vi "DisplayLogic_DrawPressStart.vi"(0 "Player":u8, 1 "ActivePixel":cluster{"h_pixel":i16, "v_pixel":i16}, 4 "PressStartPos":T1) -> (15 "PixelData":bool[](array[boolean]), 18 "Draw":bool)   [LabVIEW 2018]
uses:
  Control_GameOverGlobal.vi
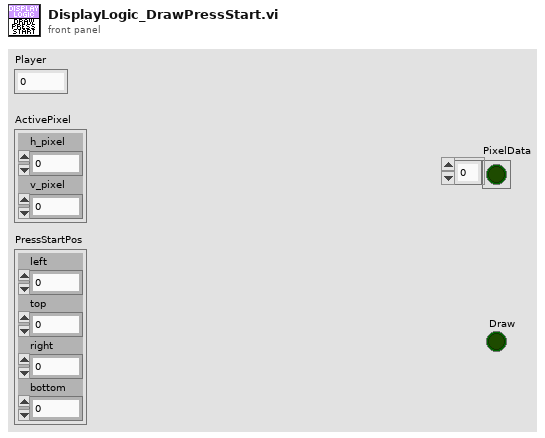
[diagram p1: front panel]
types:
  T1 = cluster{"left":i16, "top":i16, "right":i16, "bottom":i16}
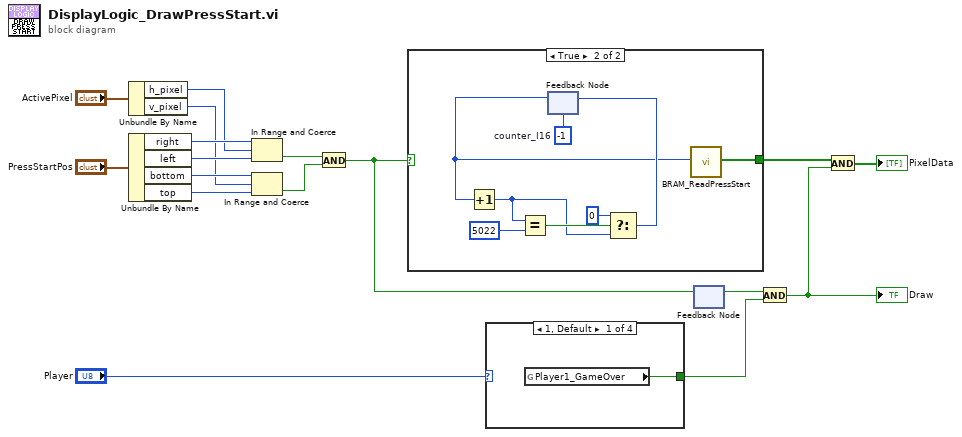
[diagram p0: block diagram]
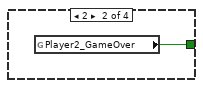
[diagram p2: hidden frame]
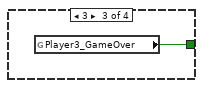
[diagram p3: hidden frame]
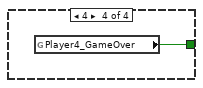
[diagram p4: hidden frame]
diagram:
  n1 = Unbundle By Name("ActivePixel") -> ("h_pixel"=w9:i16, "v_pixel"=w8:i16)
  n2 = Unbundle By Name("PressStartPos") -> ("right"=w13:i16, "left"=w17:i16, "bottom"=w11:i16, "top"=w14:i16)
  n3 = In Range and Coerce(upper limit=w13, x=w9, lower limit=w17) -> (In Range?=w16:bool)  [unwired: 1 out]
  n4 = In Range and Coerce(upper limit=w11, x=w8, lower limit=w14) -> (In Range?=w15:bool)  [unwired: 1 out]
  n5 = And(x=w16, y=w15) -> (x .and. y?=w5:bool)
  n6 = case shown="True" w5 {
    tunnel: [_ w19] -> w7
    frame False {
    }
    frame True {
      w23 = i16 -1  # counter_I16
      n7 = feedback #1(w23) -> (w20:i16)
      n8 = Increment(x=w20) -> (x+1=w18:i16)
      n9 = Equal?(x=w18, y=i16 5022) -> (x = y?=w22:bool)
      n10 = Select(t=i16 0 ("f"), s=w22, f=w18) -> (s? t:f=w25:i16)
      n11 = feedback-in #1(w25) -> ()
      n12 = call "BRAM_ReadPressStart.vi"("Address"=w20) -> ("PixelData"=w19:bool[])  [unwired: 18 in]
    }
  }
  n13 = case shown="1, Default" "Player" {
    tunnel: [w26 w27 w28 w29] -> w2
    frame 1, Default {
      n14 = global read "Control_GameOverGlobal.vi" "Player1_GameOver"() -> (w26:bool)
    }
    frame 2 {
      n15 = global read "Control_GameOverGlobal.vi" "Player2_GameOver"() -> (w27:bool)
    }
    frame 3 {
      n16 = global read "Control_GameOverGlobal.vi" "Player3_GameOver"() -> (w28:bool)
    }
    frame 4 {
      n17 = global read "Control_GameOverGlobal.vi" "Player4_GameOver"() -> (w29:bool)
    }
  }
  n18 = feedback-in #2(w5) -> ()
  n19 = feedback #2() -> (w4:bool)  [unwired: 1 in]
  n20 = And(x=w4, y=w2) -> (x .and. y?=w3:bool)
  "Draw" <- w3
  n21 = And(x=w7, y=w3) -> (x .and. y?=→"PixelData":bool[])
